vi "Joystick Control.vi"(1 "Number of Joysticks":i32=1 min=1 max=6 step=1, 2 "Mode":enum8{"Start", "Run", "Finish"}(ring)) -> (0 "Joysticks":cluster{"Buttons":bool[], "Axes":dbl[]}[](array[cluster]))   [LabVIEW 2014]
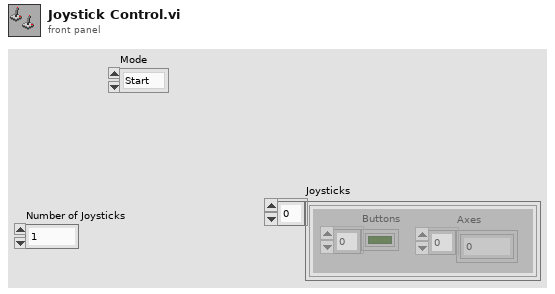
[diagram p1: front panel]
types:
  T1 = typedef "WPI_JoystickDevRef.ctl" = cluster{"Device":T2}
  T2 = typedef "WPI_JoystickDeviceEnum.ctl" = enum16{"USB 0", "USB 1", "USB 2", "USB 3", "USB 4", "USB 5"}
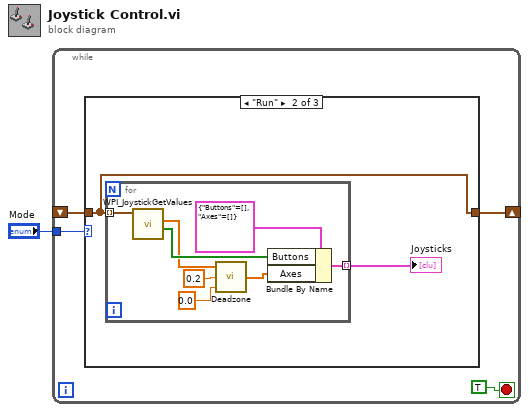
[diagram p0: block diagram]
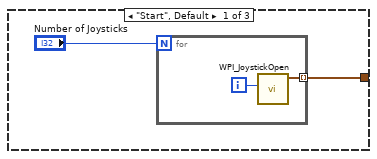
[diagram p2: hidden frame]
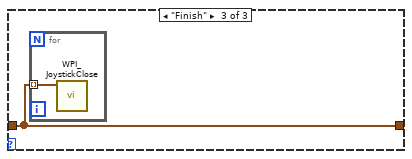
[diagram p3: hidden frame]
diagram:
  n1 = while {
    tunnel: "Mode" -> [w4]
    shift-right: [w3] -> _
    shift-left: _ -> [w2]
    stop <- TRUE stop-if-true
    n2 = case shown="\"Run\"" w4 {
      tunnel: [w6 w10 w20] -> w3
      tunnel: w2 -> [_ w10 w20]
      frame "Start", Default {
        n3 = for {
          N: "Number of Joysticks" -> [_]
          tunnel: [w9] -> w6 mode=indexing
          i -> [w8]
          n4 = call <vilib>:"WPI_JoystickOpen.vi"("JoystickDevice"=w8) -> ("JoystickDevRef"=w9:T1)  [unwired: 10 in]
        }
      }
      frame "Run" {
        n5 = for {
          tunnel: [w13] -> w11 mode=indexing
          tunnel: w10 -> [w12] mode=indexing
          n6 = call <vilib>:"WPI_JoystickGetValues.vi"("JoystickDevRef"=w12) -> ("Buttons"=w19:bool[], "Axes"=w16:dbl[])  [unwired: 6 in, 3 out]
          n7 = call "Deadzone.vi"("Default"=0.0, "Deadzone"=0.2, "Input"=w16) -> ("Output"=w15:dbl[])
          n8 = Bundle By Name(cluster=cluster{"Buttons":bool[], "Axes":dbl[]} {"Buttons"=[], "Axes"=[]} ("Joystick"), "Buttons"=w19, "Axes"=w15) -> (w13:cluster{"Buttons":bool[], "Axes":dbl[]})
        }
        "Joysticks" <- w11
      }
      frame "Finish" {
        n9 = for {
          tunnel: w20 -> [w21] mode=indexing
          n10 = call <vilib>:"WPI_JoystickClose.vi"("JoystickDevRef"=w21) -> ()  [unwired: 11 in]
        }
      }
    }
  }
